vi "Delete last one.vi"(8 "error in (no error)":errorcluster, 10 "File/Data?":bool, 11 "Directory":string[](array[string])) -> (0 "error out":errorcluster)   [LabVIEW 2017, in "File.lvlib"]
uses:
  File.lvlib
  Control/Parent path.ctl
  Control/Folder Format.ctl
  Control/File Format.ctl
  <vilib>/Utility/file.llb/Read Delimited Spreadsheet (string).vi
  <vilib>/Utility/file.llb/Write Delimited Spreadsheet (string).vi
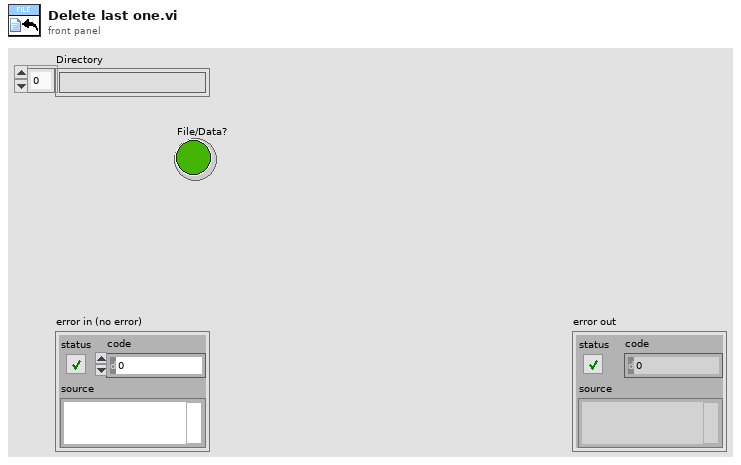
[diagram p1: front panel]
types:
  T1 = typedef "File.lvlib/Folder Format.ctl" = enum16{"None", "Folder Date", "Folder/Date"}
  T2 = typedef "File.lvlib/Parent path.ctl" = enum16{"Project", "Setting", "Log"}
  T3 = typedef "File.lvlib/File Format.ctl" = enum16{"None", "File Date", "File Time"}
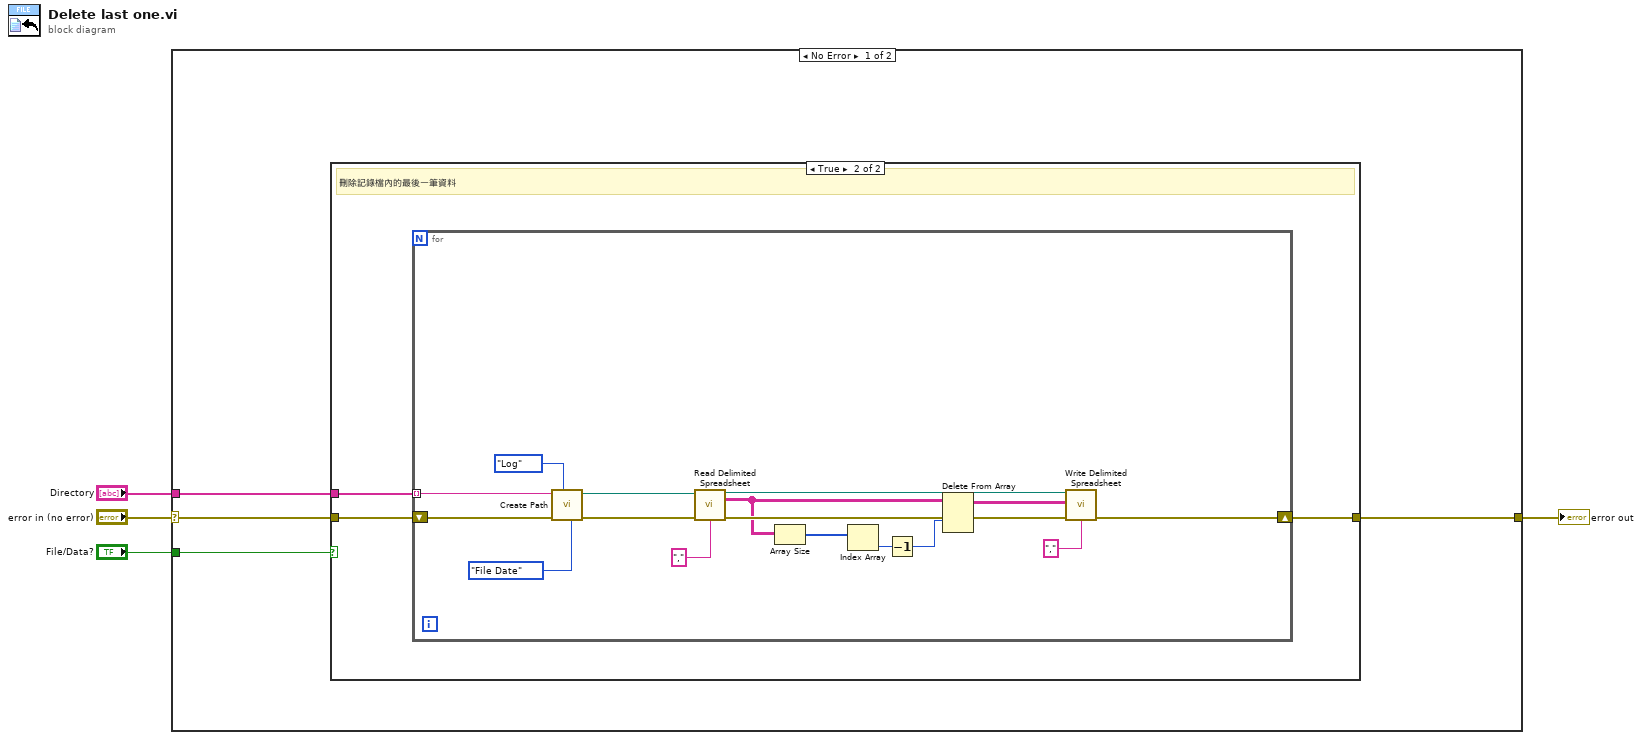
[diagram p0: block diagram]
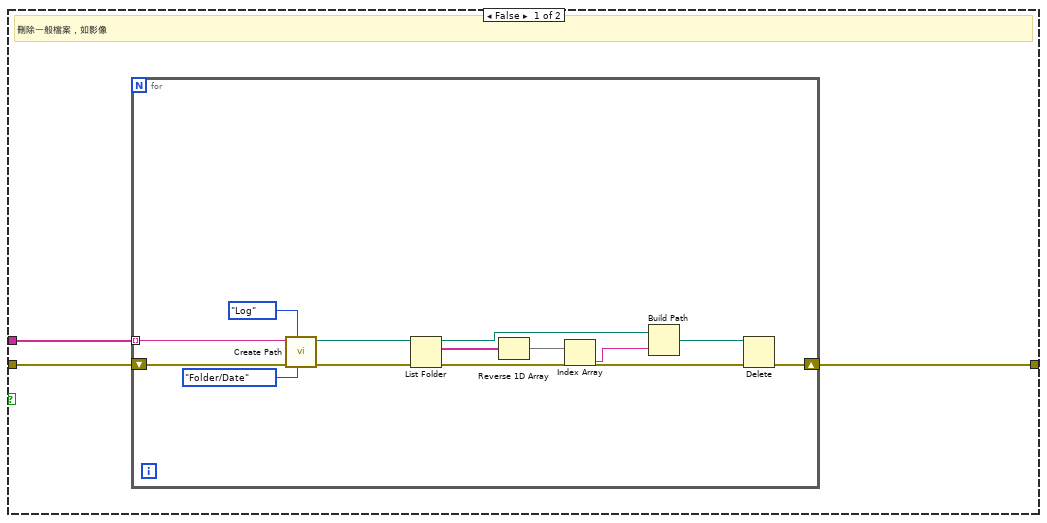
[diagram p2: hidden frame]
diagram:
  n1 = case shown="No Error" "error in (no error)" {
    selector: "error in (no error)" -> [w8 w44]
    tunnel: [w7 w44] -> w3
    tunnel: "Directory" -> [w6 _]
    tunnel: "File/Data?" -> [w5 _]
    frame No Error {
      n2 = case shown="True" w5 {
        tunnel: w8 -> [w11 w27]
        tunnel: [w10 w26] -> w7
        tunnel: w6 -> [w9 w25]
        frame False {
          # "刪除一般檔案，如影像"
          n3 = for {
            shift-right: [w15] -> w10
            shift-left: w11 -> [w24]
            tunnel: w9 -> [w14] mode=indexing
            n4 = call "Create Path.vi"("Folder Format"=Folder_Format."Folder/Date", "Parent path"=Parent_path."Log", "error in (no error)"=w24, "Directory"=w14) -> ("error out"=w23:errorcluster, "Path"=w22:path)  [unwired: 6 in]
            n5 = List Folder(path=w22, error in=w23) -> (path out=w19:path, filenames=w21:string[], error out=w17:errorcluster)  [unwired: 2 in, 1 out]
            n6 = Reverse 1D Array(array=w21) -> (reversed array=w20:string[])
            n7 = Index Array(array=w20) -> (element=w18:string)  [unwired: 1 in]
            n8 = Build Path(base path=w19, name or relative path=w18) -> (appended path=w16:path)
            n9 = Delete(path (use dialog)=w16, error in=w17) -> (error out=w15:errorcluster)  [unwired: 3 in, 2 out]
          }
        }
        frame True {
          # "刪除記錄檔內的最後一筆資料"
          n10 = for {
            shift-right: [w32] -> w26
            shift-left: w27 -> [w43]
            tunnel: w25 -> [w41] mode=indexing
            n11 = call "Create Path.vi"("File Format"=File_Format."File Date", "Parent path"=Parent_path."Log", "error in (no error)"=w43, "Directory"=w41) -> ("error out"=w42:errorcluster, "Path"=w38:path)  [unwired: 6 in]
            n12 = call-poly <vilib>:"Read Delimited Spreadsheet.vi"("file path (dialog if empty)"=w38, "error in (no error)"=w42, "delimiter (\\t)"=",") -> ("new file path (Not A Path if cancelled)"=w31:path, "all rows"=w35:string[][], "error out"=w39:errorcluster)  [unwired: 7 in, 3 out]
            n13 = Array Size(array=w35) -> (size(s)=w36:i32[])
            n14 = Index Array(array=w36) -> (element=w34:i32)  [unwired: 1 in]
            n15 = Decrement(x=w34) -> (x-1=w33:i32)
            n16 = Delete From Array(array=w35, index (row)=w33) -> (array with subset deleted=w30:string[][])  [unwired: 2 in, 1 out]
            n17 = call-poly <vilib>:"Write Delimited Spreadsheet.vi"("file path (dialog if empty)"=w31, "2D data"=w30, "error in (no error)"=w39, "delimiter (\\t)"=",") -> ("error out"=w32:errorcluster)  [unwired: 10 in, 1 out]
          }
        }
      }
    }
    frame Error {
    }
  }
  "error out" <- w3
